vi "Merge Sort String Arrays.vi"(0 "String Array A":string[](array[string]), 1 "Ignore Duplicates? (F)":bool, 3 "String Array B":string[](array[string])) -> (6 "Sorted String Array":string[](array[string]))   [LabVIEW 2013]
panel:
  out "A Index":i32
  out "B Index":i32
  out "B Count":i32
  out "A Count":i32
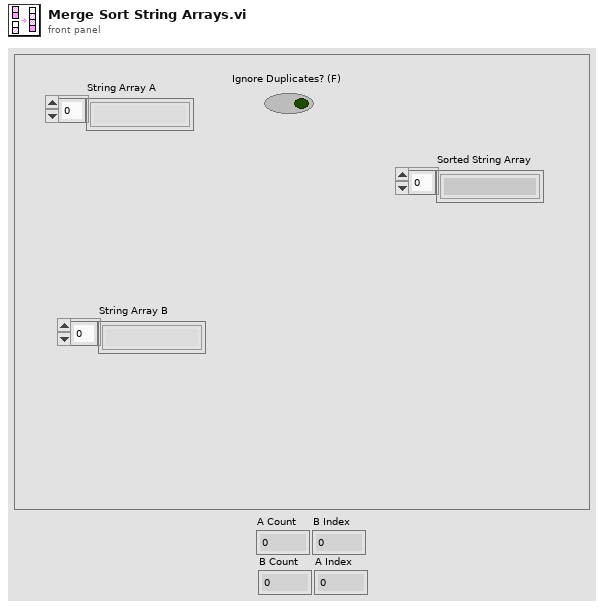
[diagram p1: front panel]
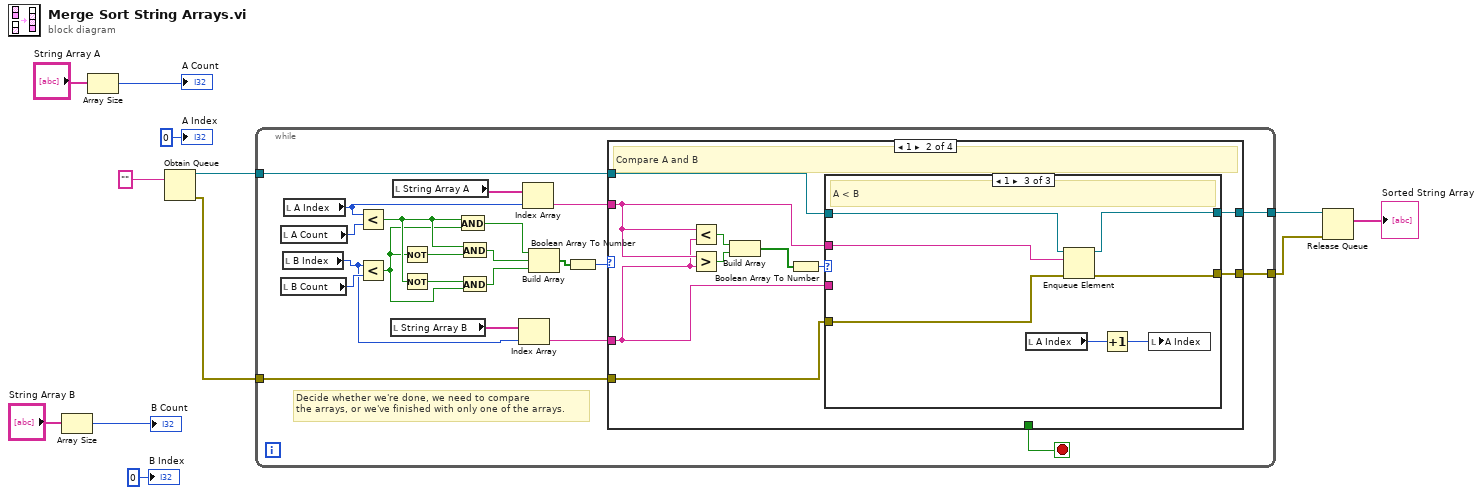
[diagram p0: block diagram]
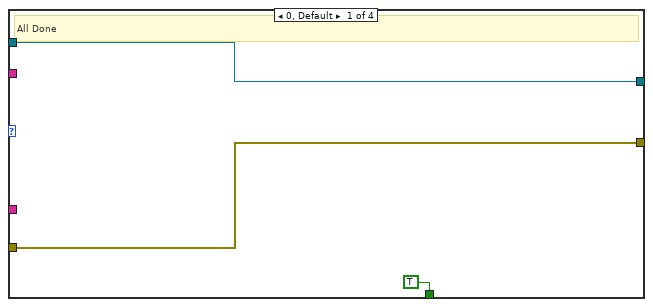
[diagram p2: hidden frame]
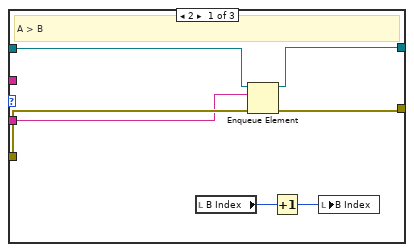
[diagram p3: hidden frame]
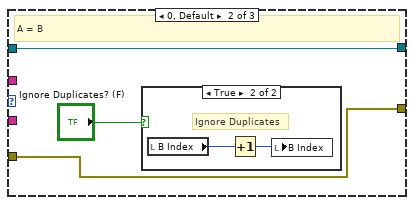
[diagram p4: hidden frame]
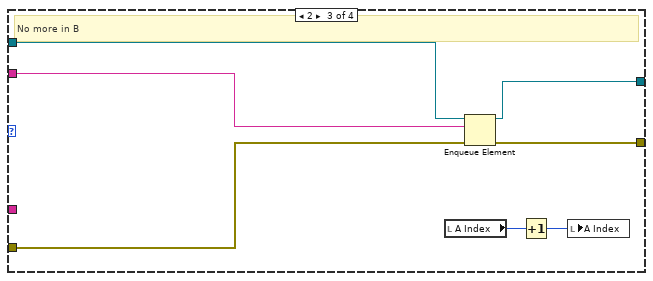
[diagram p6: hidden frame]
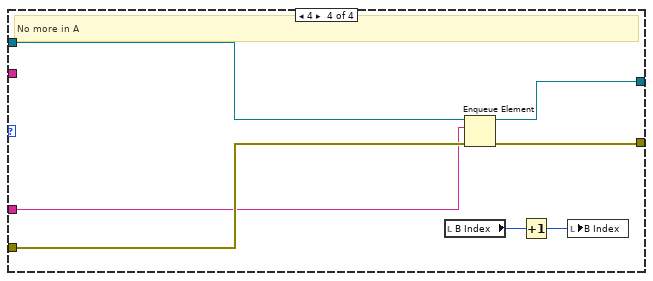
[diagram p7: hidden frame]
diagram:
  n1 = Array Size(array="String Array B") -> (size(s)=→"B Count":i32)
  n2 = Array Size(array="String Array A") -> (size(s)=→"A Count":i32)
  n3 = Obtain Queue(element data type="") -> (queue out=w11:refnum<queue>, error out=w10:errorcluster)  [unwired: 4 in, 1 out]
  n4 = while {
    tunnel: w11 -> [w23]
    tunnel: [w22] -> w3
    tunnel: [w21] -> w12
    tunnel: w10 -> [w20]
    stop <- w13 stop-if-true
    # "Decide whether we're done, we need to compare\nthe arrays, or we've finished with only one of the arrays."
    n5 = local read "A Count"() -> (w34:i32)
    n6 = local read "B Count"() -> (w33:i32)
    n7 = local read "B Index"() -> (w16:i32)
    n8 = local read "A Index"() -> (w18:i32)
    n9 = Less?(x=w18, y=w34) -> (x < y?=w30:bool)
    n10 = Less?(x=w16, y=w33) -> (x < y?=w29:bool)
    n11 = local read "String Array B"() -> (w17:string[])
    n12 = local read "String Array A"() -> (w19:string[])
    n13 = Not(x=w29) -> (.not. x?=w27:bool)
    n14 = Not(x=w30) -> (.not. x?=w26:bool)
    n15 = And(x=w30, y=w29) -> (x .and. y?=w32:bool)
    n16 = And(x=w30, y=w27) -> (x .and. y?=w31:bool)
    n17 = And(x=w26, y=w29) -> (x .and. y?=w28:bool)
    n18 = Index Array(array=w17, index=w16) -> (element=w15:string)
    n19 = Index Array(array=w19, index=w18) -> (element=w14:string)
    n20 = Build Array(w32, w31, w28) -> (w25:bool[])
    n21 = Boolean Array To Number(Boolean array=w25) -> (number=w24:u32)
    n22 = case shown="1" w24 {
      tunnel: w23 -> [w37 w47 w73 w80]
      tunnel: w14 -> [_ w39 w71 _]
      tunnel: w15 -> [_ w38 _ w78]
      tunnel: w20 -> [w36 w40 w72 w79]
      tunnel: [w36 w46 w69 w76] -> w22
      tunnel: [w37 w45 w70 w77] -> w21
      tunnel: [TRUE _ _ _] -> w13
      frame 0, Default {
        # "All Done"
      }
      frame 1 {
        # "Compare A and B"
        n23 = Less?(x=w39, y=w38) -> (x < y?=w44:bool)
        n24 = Greater?(x=w39, y=w38) -> (0:w43:bool)
        n25 = Build Array(w44, w43) -> (w42:bool[])
        n26 = Boolean Array To Number(Boolean array=w42) -> (number=w41:u32)
        n27 = case shown="1" w41 {
          tunnel: w47 -> [w54 w55 w66]
          tunnel: w39 -> [_ _ w65]
          tunnel: w38 -> [w48 _ _]
          tunnel: w40 -> [w53 w56 w64]
          tunnel: [w51 w56 w62] -> w46
          tunnel: [w52 w55 w63] -> w45
          frame 2 {
            # "A > B"
            n28 = local read "B Index"() -> (w49:i32)
            n29 = Enqueue Element(queue=w54, element=w48, error in (no error)=w53) -> (queue out=w52:refnum<queue>, error out=w51:errorcluster)  [unwired: 1 in, 1 out]
            n30 = Increment(x=w49) -> (x+1=w50:i32)
            n31 = local write "B Index"(w50) -> ()
          }
          frame 0, Default {
            # "A = B"
            n32 = case shown="True" "Ignore Duplicates? (F)" {
              frame False {
              }
              frame True {
                # "Ignore Duplicates"
                n33 = local read "B Index"() -> (w59:i32)
                n34 = Increment(x=w59) -> (x+1=w58:i32)
                n35 = local write "B Index"(w58) -> ()
              }
            }
          }
          frame 1 {
            # "A < B"
            n36 = local read "A Index"() -> (w60:i32)
            n37 = Enqueue Element(queue=w66, element=w65, error in (no error)=w64) -> (queue out=w63:refnum<queue>, error out=w62:errorcluster)  [unwired: 1 in, 1 out]
            n38 = Increment(x=w60) -> (x+1=w61:i32)
            n39 = local write "A Index"(w61) -> ()
          }
        }
      }
      frame 2 {
        # "No more in B"
        n40 = local read "A Index"() -> (w67:i32)
        n41 = Enqueue Element(queue=w73, element=w71, error in (no error)=w72) -> (queue out=w70:refnum<queue>, error out=w69:errorcluster)  [unwired: 1 in, 1 out]
        n42 = Increment(x=w67) -> (x+1=w68:i32)
        n43 = local write "A Index"(w68) -> ()
      }
      frame 4 {
        # "No more in A"
        n44 = local read "B Index"() -> (w74:i32)
        n45 = Enqueue Element(queue=w80, element=w78, error in (no error)=w79) -> (queue out=w77:refnum<queue>, error out=w76:errorcluster)  [unwired: 1 in, 1 out]
        n46 = Increment(x=w74) -> (x+1=w75:i32)
        n47 = local write "B Index"(w75) -> ()
      }
    }
  }
  n48 = Release Queue(queue=w12, error in (no error)=w3) -> (remaining elements=→"Sorted String Array":string[])  [unwired: 1 in, 2 out]
  "A Index" <- 0 ("A Index")
  "B Index" <- 0 ("B Index")
